vi "Gas Controller.vi"() -> ()   [LabVIEW 2013]
uses:
  Program Files/National Instruments/LabVIEW 2018/instr.lib/MultiGasController/647 Multi Gas Controller.llb/647 Open/Close Valve .vi
  <vilib>/MakerHub/LINX/LMH-LINX.lvlib
  <vilib>/MakerHub/LINX/Public/Sensors/Motion/Servo/Servo.lvlib
  <vilib>/Instr/_visa.llb/VISA Configure Serial Port (Instr).vi
  <vilib>/MakerHub/LINX/Public/Sensors/Motion/Servo/Servo Set Pulse Width One Channel.vi
  <vilib>/MakerHub/LINX/Public/Utilities/Open Serial.vi
  <vilib>/MakerHub/LINX/Public/Sensors/Motion/Servo/Servo Open One Channel.vi
  <vilib>/MakerHub/LINX/Public/Sensors/Motion/Servo/Servo Close One Channel.vi
  <vilib>/ErrorRing/Error Ring.xnode
  <vilib>/Utility/error.llb/Error Cluster From Error Code.vi
panel:
  out "MFC 8 Flow":dbl=-0.0
  out "MFC 7 Flow":dbl=-0.0
  out "MFC 6 Flow":dbl
  out "MFC 5 Flow":dbl=-0.094
  out "MFC 4 Flow":dbl=-0.303
  out "MFC 3 Flow":dbl=0.061
  out "MFC 2 Flow":dbl=-0.18
  out "MFC 1 Flow":dbl=10.022499999999999
  in  "Servo Channel":u8=11
  in  "On Position":dbl=860.0
  in  "Off Position":dbl=1900.0
  in  "Arduino Port":refnum<visa-resource-name>="COM7"
  in  "GCF 8":dbl=1.0
  in  "GCF 7":dbl=1.0
  in  "GCF 6":dbl=0.7
  in  "MFC 8 Size":dbl=1.0
  in  "MFC 7 Size":dbl=1.0
  in  "MFC 6 Size":dbl=50.0
  out "MFC 8 Status":bool
  out "MFC 7 Status":bool
  out "MFC 6 Status":bool
  in  "MFC 7":bool
  in  "MFC 8":bool
  in  "MFC 6: CO2":bool
  in  "MFC 8 set point":dbl
  in  "MFC 7 set point":dbl
  in  "MFC 6 set point":dbl
  in  "GCF 5":dbl=0.94
  in  "GCF 4":dbl=1.01
  in  "GCF 3":dbl=1.22
  in  "GCF 2":dbl=0.9
  in  "GCF 1":dbl=0.95
  in  "MFC 5 Size":dbl=100.0
  in  "MFC 4 Size":dbl=50.0
  in  "MFC 3 Size":dbl=50.0
  in  "MFC 2 Size":dbl=100.0
  in  "MFC 1 Size":dbl=50.0
  in  "stop":bool
  out "MFC 5 Status":bool
  out "MFC 4 Status":bool
  out "MFC 1 Status":bool=TRUE
  out "MFC 2 Status":bool
  out "MFC 3 Status":bool
  in  "MFC 2: N2":bool
  in  "MFC 2 set point":dbl=50.0
  in  "MFC 4: H2":bool
  in  "MFC 5: N2 (Wet)":bool
  in  "MFC 3: O2":bool
  in  "MFC 1: N2 to Microbalance":bool=TRUE
  in  "MFC 5 set point":dbl=48.5
  in  "MFC 4 set point":dbl=50.0
  in  "MFC 3 set point":dbl=50.0
  in  "MFC 1  set point":dbl=10.0
  in  "MKS Controller Port":refnum<visa-resource-name>="COM5"
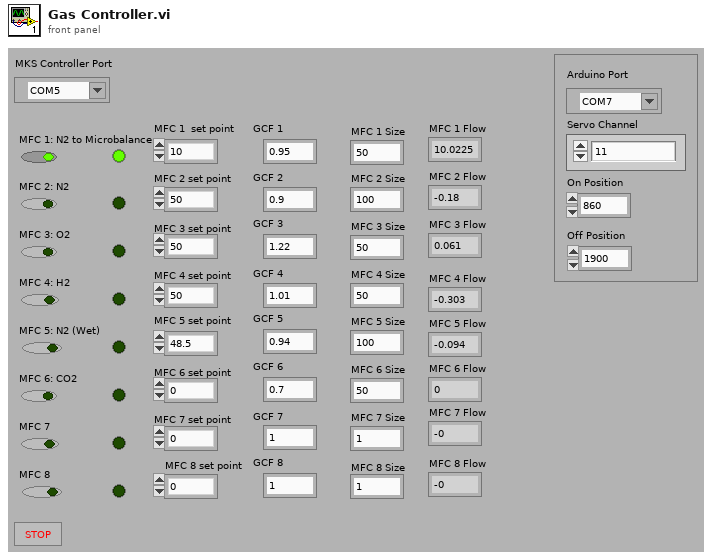
[diagram p1: front panel]
types:
  T1 = typedef "LMH-LINX.lvlib/LINX Ref.ctl" = cluster{"IO":T2, "Interface":T3, "LINX Device Config":T4}
  T2 = typedef "LMH-LINX.lvlib/Platform.ctl" = enum16{"Remote", "Local"}
  T3 = typedef "LMH-LINX.lvlib/Interface.ctl" = enum16{"Serial", "TCP"}
  T4 = typedef "LMH-LINX.lvlib/Device.lvlib/LINX Device Config.ctl" = cluster{"Interface":T3, "COM Port":refnum<visa-resource-name>, "TCP Configuration":T5, "Device Family":u8, "Device ID":u8, "Device Name":string, "TCP Ref":refnum<k5>, "Channels":T6}
  T5 = typedef "LMH-LINX.lvlib/Device.lvlib/TCP Config.ctl" = cluster{"IP Address":string, "Port":u16}
  T6 = typedef "LMH-LINX.lvlib/Channels.ctl" = cluster{"DI":u8[], "DO":u8[], "AI":u8[], "AO":u8[], "PWM":u8[], "QE":u8[], "UART":u8[], "I2C 2":u8[], "SPI":u8[], "CAN":u8[], "Servo":u8[], "AI Ref (V)":dbl, "AI Resolution (Bits)":u8, "AO Ref (V)":dbl, "AO Resolution (Bits)":u8}
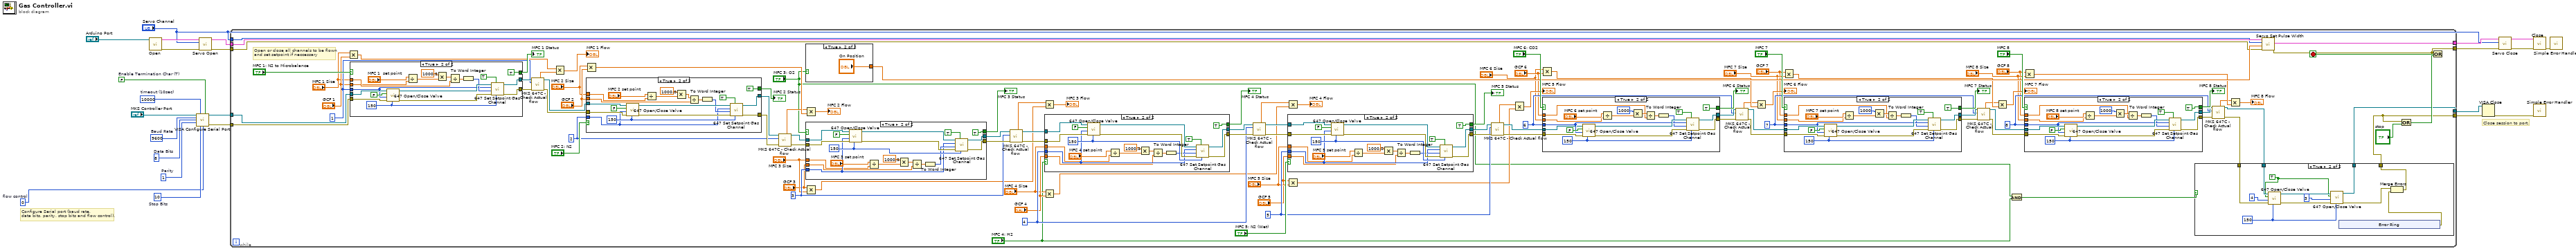
[diagram p0: block diagram]
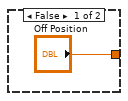
[diagram p3: hidden frame]
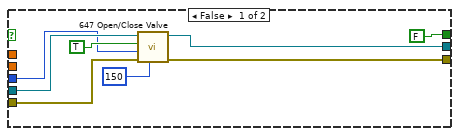
[diagram p4: hidden frame]
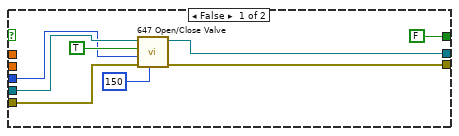
[diagram p5: hidden frame]
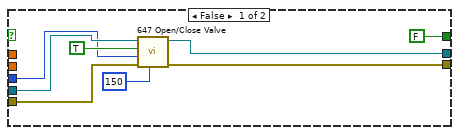
[diagram p6: hidden frame]
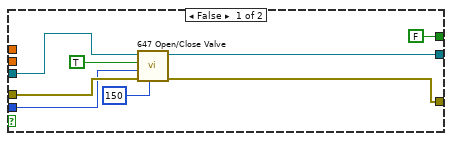
[diagram p7: hidden frame]
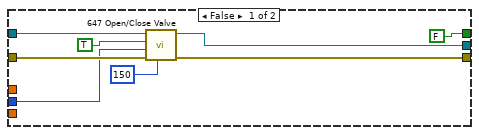
[diagram p8: hidden frame]
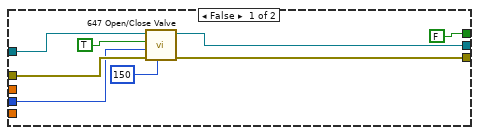
[diagram p9: hidden frame]
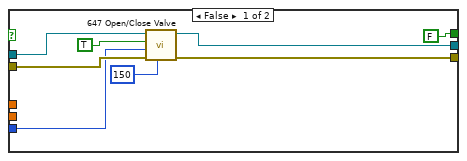
[diagram p10: hidden frame]
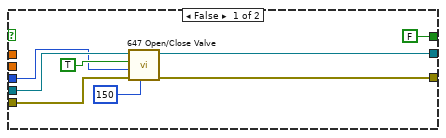
[diagram p11: hidden frame]
diagram:
  w17 = 0  # flow control
  w18 = 10  # Stop Bits
  w19 = 1  # Parity
  w20 = 8  # Data Bits
  w21 = 9600  # Baud Rate
  w22 = FALSE  # Enable Termination Char (T)
  w23 = u32 10000  # timeout (10sec)
  # "Close session to port."
  # "Configure Serial port (baud rate,\ndata bits, parity, stop bits and flow control)."
  n1 = call-poly <vilib>:"Open.vi"("Serial Port"="Arduino Port") -> ("Error Out"=w7:errorcluster, "LINX Resource"=w8:T1)  [unwired: 8 in, 1 out]
  n2 = call-poly "VISA Configure Serial Port"("VISA resource name"="MKS Controller Port", "timeout (10sec)"=w23, "Enable Termination\nChar (T)"=w22, "baud rate (9600)"=w21, "data bits (8)"=w20, "parity (0:none)"=w19, "stop bits (10: 1 bit)"=w18, "flow control (0:none)"=w17) -> ("VISA resource name out"=w16:refnum<visa-resource-name>, "error out"=w15:errorcluster)  [unwired: 6 in]
  n3 = call-poly <vilib>:"Servo Open.vi"("Error In"=w7, "Servo Channel"="Servo Channel", "LINX Resource"=w8) -> ("Error Out"=w4:errorcluster, "LINX Resource"=w5:T1)  [unwired: 7 in]
  n4 = while {
    tunnel: w16 -> [w126]
    tunnel: w15 -> [w125]
    tunnel: [w25] -> w13
    tunnel: [w26] -> w12
    tunnel: w5 -> [w117]
    tunnel: w4 -> [w116]
    tunnel: [w33] -> w3
    tunnel: [w115] -> w2
    tunnel: "Servo Channel" -> [w114]
    stop <- w35 stop-if-true
    w42 = 8
    w50 = 7
    w59 = 6
    w89 = 3
    w79 = 4
    w69 = 5
    w99 = 2
    w109 = 1
    # "Open or close all channels to be flown\nand set setpoint if neccessary"
    n5 = Multiply(x="MFC 1 Size", y="GCF 1") -> (x*y=w108:dbl)
    n6 = case shown="True" "MFC 1: N2 to Microbalance" {
      tunnel: w125 -> [w348 w371]
      tunnel: [w349 w366] -> w111
      tunnel: w126 -> [w351 w370]
      tunnel: [w350 w367] -> w113
      tunnel: w109 -> [w347 w357]
      tunnel: [FALSE TRUE] -> w129
      tunnel: "GCF 1" -> [_ w354]
      tunnel: "MFC 1 Size" -> [_ w353]
      frame False {
        n7 = call "647 Open/Close Valve .vi"("ms Wartezeit"=u32 150, "error in (no error)"=w348, "Channel number"=w347, "OPEN / CLOSE"=TRUE, "VISA session"=w351) -> ("error out"=w349:errorcluster, "dup VISA session"=w350:refnum<visa-resource-name>)  [unwired: 4 in, 1 out]
      }
      frame True {
        w364 = 150
        n8 = call "647 Open/Close Valve .vi"("ms Wartezeit"=w364, "error in (no error)"=w371, "Channel number"=w357, "OPEN / CLOSE"=FALSE, "VISA session"=w370) -> ("error out"=w365:errorcluster, "dup VISA session"=w368:refnum<visa-resource-name>)  [unwired: 4 in, 1 out]
        n9 = Divide(x="MFC 1  set point", y=w353) -> (x/y=w359:dbl)
        n10 = Multiply(x=1000.0, y=w359) -> (x*y=w358:dbl)
        n11 = Divide(x=w358, y=w354) -> (x/y=w355:dbl)
        n12 = To Word Integer(number=w355) -> (16bit integer=w362:i16)
        n13 = call "647 Set Setpoint Gas Channel.vi"("ms Wartezeit"=w364, "Read / Write"=TRUE, "error in (no error)"=w365, "Setpoint 0..1100\n0.1% F.S. MFC"=w362, "Channel number"=w357, "VISA session"=w368) -> ("error out"=w366:errorcluster, "dup VISA session"=w367:refnum<visa-resource-name>)  [unwired: 3 in, 1 out]
      }
    }
    "MFC 1 Status" <- w129
    n14 = call "MKS 647C - Check Actual flow.vi"("error in (no error)"=w111, "Channel"=w109, "VISA resource name (IN)"=w113) -> ("error out"=w110:errorcluster, "VISA resource name (OUT)"=w112:refnum<visa-resource-name>, "Flow value"=w106:dbl)  [unwired: 6 in]
    n15 = Multiply(x=w108, y=w106) -> (x*y=→"MFC 1 Flow":dbl)
    n16 = Multiply(x="MFC 2 Size", y="GCF 2") -> (x*y=w97:dbl)
    n17 = case shown="True" "MFC 2: N2" {
      tunnel: w112 -> [w242 w263]
      tunnel: w110 -> [w241 w262]
      tunnel: [w240 w259] -> w100
      tunnel: [w239 w258] -> w103
      tunnel: w99 -> [w238 w252]
      tunnel: [FALSE TRUE] -> w130
      tunnel: "MFC 2 Size" -> [_ w246]
      tunnel: "GCF 2" -> [_ w245]
      frame False {
        n18 = call "647 Open/Close Valve .vi"("ms Wartezeit"=u32 150, "error in (no error)"=w241, "Channel number"=w238, "OPEN / CLOSE"=TRUE, "VISA session"=w242) -> ("error out"=w240:errorcluster, "dup VISA session"=w239:refnum<visa-resource-name>)  [unwired: 4 in, 1 out]
      }
      frame True {
        w256 = 150
        n19 = call "647 Open/Close Valve .vi"("ms Wartezeit"=w256, "error in (no error)"=w262, "Channel number"=w252, "OPEN / CLOSE"=FALSE, "VISA session"=w263) -> ("error out"=w260:errorcluster, "dup VISA session"=w257:refnum<visa-resource-name>)  [unwired: 4 in, 1 out]
        n20 = Divide(x="MFC 2 set point", y=w246) -> (x/y=w251:dbl)
        n21 = Multiply(x=1000.0, y=w251) -> (x*y=w247:dbl)
        n22 = Divide(x=w247, y=w245) -> (x/y=w248:dbl)
        n23 = To Word Integer(number=w248) -> (16bit integer=w254:i16)
        n24 = call "647 Set Setpoint Gas Channel.vi"("ms Wartezeit"=w256, "Read / Write"=TRUE, "error in (no error)"=w260, "Setpoint 0..1100\n0.1% F.S. MFC"=w254, "Channel number"=w252, "VISA session"=w257) -> ("error out"=w259:errorcluster, "dup VISA session"=w258:refnum<visa-resource-name>)  [unwired: 3 in, 1 out]
      }
    }
    "MFC 2 Status" <- w130
    n25 = call "MKS 647C - Check Actual flow.vi"("error in (no error)"=w100, "Channel"=w99, "VISA resource name (IN)"=w103) -> ("error out"=w101:errorcluster, "VISA resource name (OUT)"=w102:refnum<visa-resource-name>, "Flow value"=w96:dbl)  [unwired: 6 in]
    n26 = Multiply(x=w96, y=w97) -> (x*y=→"MFC 2 Flow":dbl)
    n27 = Multiply(x="GCF 3", y="MFC 3 Size") -> (x*y=w87:dbl)
    n28 = case shown="True" "MFC 3: O2" {
      tunnel: ["Off Position" "On Position"] -> w118
      frame False {
      }
      frame True {
      }
    }
    n29 = case shown="True" "MFC 3: O2" {
      tunnel: w101 -> [w323 w344]
      tunnel: [w324 w338] -> w92
      tunnel: w102 -> [w322 w343]
      tunnel: [w325 w341] -> w91
      tunnel: w89 -> [w320 w332]
      tunnel: [FALSE TRUE] -> w131
      tunnel: "MFC 3 Size" -> [_ w327]
      tunnel: "GCF 3" -> [_ w326]
      frame False {
        n30 = call "647 Open/Close Valve .vi"("ms Wartezeit"=u32 150, "error in (no error)"=w323, "Channel number"=w320, "OPEN / CLOSE"=TRUE, "VISA session"=w322) -> ("error out"=w324:errorcluster, "dup VISA session"=w325:refnum<visa-resource-name>)  [unwired: 4 in, 1 out]
      }
      frame True {
        w337 = 150
        n31 = call "647 Open/Close Valve .vi"("ms Wartezeit"=w337, "error in (no error)"=w344, "Channel number"=w332, "OPEN / CLOSE"=FALSE, "VISA session"=w343) -> ("error out"=w339:errorcluster, "dup VISA session"=w340:refnum<visa-resource-name>)  [unwired: 4 in, 1 out]
        n32 = Divide(x="MFC 3 set point", y=w327) -> (x/y=w335:dbl)
        n33 = Multiply(x=1000.0, y=w335) -> (x*y=w328:dbl)
        n34 = Divide(x=w328, y=w326) -> (x/y=w329:dbl)
        n35 = To Word Integer(number=w329) -> (16bit integer=w334:i16)
        n36 = call "647 Set Setpoint Gas Channel.vi"("ms Wartezeit"=w337, "Read / Write"=TRUE, "error in (no error)"=w339, "Setpoint 0..1100\n0.1% F.S. MFC"=w334, "Channel number"=w332, "VISA session"=w340) -> ("error out"=w338:errorcluster, "dup VISA session"=w341:refnum<visa-resource-name>)  [unwired: 3 in, 1 out]
      }
    }
    "MFC 3 Status" <- w131
    n37 = call "MKS 647C - Check Actual flow.vi"("error in (no error)"=w92, "Channel"=w89, "VISA resource name (IN)"=w91) -> ("error out"=w93:errorcluster, "VISA resource name (OUT)"=w90:refnum<visa-resource-name>, "Flow value"=w84:dbl)  [unwired: 6 in]
    n38 = Multiply(x=w84, y=w87) -> (x*y=→"MFC 3 Flow":dbl)
    n39 = Multiply(x="MFC 4 Size", y="GCF 4") -> (x*y=w77:dbl)
    n40 = case shown="True" "MFC 4: H2" {
      tunnel: w93 -> [w298 w316]
      tunnel: [w297 w312] -> w81
      tunnel: w90 -> [w296 w317]
      tunnel: [w295 w313] -> w80
      tunnel: [FALSE TRUE] -> w128
      tunnel: w79 -> [w291 w303]
      tunnel: "MFC 4 Size" -> [_ w300]
      tunnel: "GCF 4" -> [_ w299]
      frame False {
        n41 = call "647 Open/Close Valve .vi"("ms Wartezeit"=u32 150, "error in (no error)"=w298, "Channel number"=w291, "OPEN / CLOSE"=TRUE, "VISA session"=w296) -> ("error out"=w297:errorcluster, "dup VISA session"=w295:refnum<visa-resource-name>)  [unwired: 4 in, 1 out]
      }
      frame True {
        w310 = u32 150
        n42 = call "647 Open/Close Valve .vi"("ms Wartezeit"=w310, "error in (no error)"=w316, "Channel number"=w303, "OPEN / CLOSE"=FALSE, "VISA session"=w317) -> ("error out"=w311:errorcluster, "dup VISA session"=w314:refnum<visa-resource-name>)  [unwired: 4 in, 1 out]
        n43 = Divide(x="MFC 4 set point", y=w300) -> (x/y=w308:dbl)
        n44 = Multiply(x=1000.0, y=w308) -> (x*y=w301:dbl)
        n45 = Divide(x=w301, y=w299) -> (x/y=w302:dbl)
        n46 = To Word Integer(number=w302) -> (16bit integer=w307:i16)
        n47 = call "647 Set Setpoint Gas Channel.vi"("ms Wartezeit"=w310, "Read / Write"=TRUE, "error in (no error)"=w311, "Setpoint 0..1100\n0.1% F.S. MFC"=w307, "Channel number"=w303, "VISA session"=w314) -> ("error out"=w312:errorcluster, "dup VISA session"=w313:refnum<visa-resource-name>)  [unwired: 3 in, 1 out]
      }
    }
    "MFC 4 Status" <- w128
    n48 = call "MKS 647C - Check Actual flow.vi"("error in (no error)"=w81, "Channel"=w79, "VISA resource name (IN)"=w80) -> ("error out"=w82:errorcluster, "VISA resource name (OUT)"=w83:refnum<visa-resource-name>, "Flow value"=w74:dbl)  [unwired: 6 in]
    n49 = Multiply(x=w74, y=w77) -> (x*y=→"MFC 4 Flow":dbl)
    n50 = Multiply(x="GCF 5", y="MFC 5 Size") -> (x*y=w67:dbl)
    n51 = case shown="True" "MFC 5: N2 (Wet)" {
      tunnel: w82 -> [w271 w289]
      tunnel: w83 -> [w270 w290]
      tunnel: [FALSE TRUE] -> w127
      tunnel: w69 -> [w266 w278]
      tunnel: [w264 w275] -> w73
      tunnel: [w265 w274] -> w70
      tunnel: "GCF 5" -> [_ w273]
      tunnel: "MFC 5 Size" -> [_ w272]
      frame False {
        n52 = call "647 Open/Close Valve .vi"("ms Wartezeit"=u32 150, "error in (no error)"=w271, "Channel number"=w266, "OPEN / CLOSE"=TRUE, "VISA session"=w270) -> ("error out"=w265:errorcluster, "dup VISA session"=w264:refnum<visa-resource-name>)  [unwired: 4 in, 1 out]
      }
      frame True {
        w285 = u32 150
        n53 = call "647 Open/Close Valve .vi"("ms Wartezeit"=w285, "error in (no error)"=w289, "Channel number"=w278, "OPEN / CLOSE"=FALSE, "VISA session"=w290) -> ("error out"=w286:errorcluster, "dup VISA session"=w287:refnum<visa-resource-name>)  [unwired: 4 in, 1 out]
        n54 = Divide(x="MFC 5 set point", y=w272) -> (x/y=w283:dbl)
        n55 = Multiply(x=1000.0, y=w283) -> (x*y=w277:dbl)
        n56 = Divide(x=w277, y=w273) -> (x/y=w276:dbl)
        n57 = To Word Integer(number=w276) -> (16bit integer=w282:i16)
        n58 = call "647 Set Setpoint Gas Channel.vi"("ms Wartezeit"=w285, "Read / Write"=TRUE, "error in (no error)"=w286, "Setpoint 0..1100\n0.1% F.S. MFC"=w282, "Channel number"=w278, "VISA session"=w287) -> ("error out"=w274:errorcluster, "dup VISA session"=w275:refnum<visa-resource-name>)  [unwired: 3 in, 1 out]
      }
    }
    "MFC 5 Status" <- w127
    n59 = call "MKS 647C - Check Actual flow.vi"("error in (no error)"=w70, "Channel"=w69, "VISA resource name (IN)"=w73) -> ("error out"=w71:errorcluster, "VISA resource name (OUT)"=w72:refnum<visa-resource-name>, "Flow value"=w66:dbl)  [unwired: 6 in]
    n60 = Multiply(x=w66, y=w67) -> (x*y=→"MFC 5 Flow":dbl)
    n61 = Multiply(x="MFC 6 Size", y="GCF 6") -> (x*y=w58:dbl)
    n62 = case shown="True" "MFC 6: CO2" {
      tunnel: [FALSE TRUE] -> w123
      tunnel: [w216 w231] -> w61
      tunnel: [w214 w230] -> w60
      tunnel: w59 -> [w212 w229]
      tunnel: w72 -> [w215 w227]
      tunnel: w71 -> [w217 w226]
      tunnel: "GCF 6" -> [_ w219]
      tunnel: "MFC 6 Size" -> [_ w218]
      frame False {
        n63 = call "647 Open/Close Valve .vi"("ms Wartezeit"=150, "error in (no error)"=w217, "Channel number"=w212, "OPEN / CLOSE"=TRUE, "VISA session"=w215) -> ("error out"=w216:errorcluster, "dup VISA session"=w214:refnum<visa-resource-name>)  [unwired: 4 in, 1 out]
      }
      frame True {
        w228 = 150
        n64 = call "647 Open/Close Valve .vi"("ms Wartezeit"=w228, "error in (no error)"=w226, "Channel number"=w229, "OPEN / CLOSE"=FALSE, "VISA session"=w227) -> ("error out"=w234:errorcluster, "dup VISA session"=w233:refnum<visa-resource-name>)  [unwired: 4 in, 1 out]
        n65 = Divide(x="MFC 6 set point", y=w218) -> (x/y=w224:dbl)
        n66 = Multiply(x=1000, y=w224) -> (x*y=w220:dbl)
        n67 = Divide(x=w220, y=w219) -> (x/y=w222:dbl)
        n68 = To Word Integer(number=w222) -> (16bit integer=w221:i16)
        n69 = call "647 Set Setpoint Gas Channel.vi"("ms Wartezeit"=w228, "Read / Write"=TRUE, "error in (no error)"=w234, "Setpoint 0..1100\n0.1% F.S. MFC"=w221, "Channel number"=w229, "VISA session"=w233) -> ("error out"=w231:errorcluster, "dup VISA session"=w230:refnum<visa-resource-name>)  [unwired: 3 in, 1 out]
      }
    }
    "MFC 6 Status" <- w123
    n70 = call "MKS 647C - Check Actual flow.vi"("error in (no error)"=w61, "Channel"=w59, "VISA resource name (IN)"=w60) -> ("error out"=w62:errorcluster, "VISA resource name (OUT)"=w63:refnum<visa-resource-name>, "Flow value"=w54:dbl)  [unwired: 6 in]
    n71 = Multiply(x=w54, y=w58) -> (x*y=→"MFC 6 Flow":dbl)
    n72 = Multiply(x="GCF 7", y="MFC 7 Size") -> (x*y=w49:dbl)
    n73 = case shown="True" "MFC 7" {
      tunnel: [FALSE TRUE] -> w122
      tunnel: w62 -> [w190 w204]
      tunnel: [w189 w203] -> w51
      tunnel: w63 -> [w188 w202]
      tunnel: [w187 w201] -> w53
      tunnel: w50 -> [w185 w200]
      tunnel: "MFC 7 Size" -> [_ w192]
      tunnel: "GCF 7" -> [_ w191]
      frame False {
        n74 = call "647 Open/Close Valve .vi"("ms Wartezeit"=150, "error in (no error)"=w190, "Channel number"=w185, "OPEN / CLOSE"=TRUE, "VISA session"=w188) -> ("error out"=w189:errorcluster, "dup VISA session"=w187:refnum<visa-resource-name>)  [unwired: 4 in, 1 out]
      }
      frame True {
        w199 = 150
        n75 = call "647 Open/Close Valve .vi"("ms Wartezeit"=w199, "error in (no error)"=w204, "Channel number"=w200, "OPEN / CLOSE"=FALSE, "VISA session"=w202) -> ("error out"=w207:errorcluster, "dup VISA session"=w208:refnum<visa-resource-name>)  [unwired: 4 in, 1 out]
        n76 = Divide(x="MFC 7 set point", y=w192) -> (x/y=w197:dbl)
        n77 = Multiply(x=1000, y=w197) -> (x*y=w193:dbl)
        n78 = Divide(x=w193, y=w191) -> (x/y=w195:dbl)
        n79 = To Word Integer(number=w195) -> (16bit integer=w194:i16)
        n80 = call "647 Set Setpoint Gas Channel.vi"("ms Wartezeit"=w199, "Read / Write"=TRUE, "error in (no error)"=w207, "Setpoint 0..1100\n0.1% F.S. MFC"=w194, "Channel number"=w200, "VISA session"=w208) -> ("error out"=w203:errorcluster, "dup VISA session"=w201:refnum<visa-resource-name>)  [unwired: 3 in, 1 out]
      }
    }
    "MFC 7 Status" <- w122
    n81 = call "MKS 647C - Check Actual flow.vi"("error in (no error)"=w51, "Channel"=w50, "VISA resource name (IN)"=w53) -> ("error out"=w52:errorcluster, "VISA resource name (OUT)"=w29:refnum<visa-resource-name>, "Flow value"=w46:dbl)  [unwired: 6 in]
    n82 = Multiply(x=w46, y=w49) -> (x*y=→"MFC 7 Flow":dbl)
    n83 = And(x="MFC 3: O2", y="MFC 4: H2") -> (x .and. y?=w32:bool)
    n84 = Multiply(x="GCF 8", y="MFC 8 Size") -> (x*y=w41:dbl)
    n85 = case shown="True" "MFC 8" {
      tunnel: [FALSE TRUE] -> w121
      tunnel: w52 -> [w163 w177]
      tunnel: w29 -> [w161 w176]
      tunnel: w42 -> [w158 w175]
      tunnel: [w162 w173] -> w44
      tunnel: [w160 w167] -> w43
      tunnel: "MFC 8 Size" -> [_ w165]
      tunnel: "GCF 8" -> [_ w164]
      frame False {
        n86 = call "647 Open/Close Valve .vi"("ms Wartezeit"=150, "error in (no error)"=w163, "Channel number"=w158, "OPEN / CLOSE"=TRUE, "VISA session"=w161) -> ("error out"=w162:errorcluster, "dup VISA session"=w160:refnum<visa-resource-name>)  [unwired: 4 in, 1 out]
      }
      frame True {
        w174 = 150
        n87 = call "647 Open/Close Valve .vi"("ms Wartezeit"=w174, "error in (no error)"=w177, "Channel number"=w175, "OPEN / CLOSE"=FALSE, "VISA session"=w176) -> ("error out"=w180:errorcluster, "dup VISA session"=w181:refnum<visa-resource-name>)  [unwired: 4 in, 1 out]
        n88 = Divide(x="MFC 8 set point", y=w165) -> (x/y=w171:dbl)
        n89 = Multiply(x=1000, y=w171) -> (x*y=w166:dbl)
        n90 = Divide(x=w166, y=w164) -> (x/y=w169:dbl)
        n91 = To Word Integer(number=w169) -> (16bit integer=w168:i16)
        n92 = call "647 Set Setpoint Gas Channel.vi"("ms Wartezeit"=w174, "Read / Write"=TRUE, "error in (no error)"=w180, "Setpoint 0..1100\n0.1% F.S. MFC"=w168, "Channel number"=w175, "VISA session"=w181) -> ("error out"=w173:errorcluster, "dup VISA session"=w167:refnum<visa-resource-name>)  [unwired: 3 in, 1 out]
      }
    }
    "MFC 8 Status" <- w121
    n93 = call "MKS 647C - Check Actual flow.vi"("error in (no error)"=w44, "Channel"=w42, "VISA resource name (IN)"=w43) -> ("error out"=w28:errorcluster, "VISA resource name (OUT)"=w27:refnum<visa-resource-name>, "Flow value"=w37:dbl)  [unwired: 6 in]
    n94 = case shown="True" w32 {
      tunnel: w27 -> [w136 w146]
      tunnel: [w136 w145] -> w26
      tunnel: [w135 w137] -> w25
      tunnel: w28 -> [w135 w144]
      frame False {
      }
      frame True {
        w142 = TRUE
        w143 = 150
        n95 = call "647 Open/Close Valve .vi"("ms Wartezeit"=w143, "error in (no error)"=w144, "Channel number"=4, "OPEN / CLOSE"=w142, "VISA session"=w146) -> ("error out"=w148:errorcluster, "dup VISA session"=w147:refnum<visa-resource-name>)  [unwired: 4 in, 1 out]
        n96 = call "647 Open/Close Valve .vi"("ms Wartezeit"=w143, "error in (no error)"=w148, "Channel number"=3, "OPEN / CLOSE"=w142, "VISA session"=w147) -> ("error out"=w138:errorcluster, "dup VISA session"=w145:refnum<visa-resource-name>)  [unwired: 4 in, 1 out]
        n97 = xnode "Error Ring"() -> ("error out"=w139:errorcluster)
        n98 = Merge Errors(w138, w139) -> (w137:errorcluster)
      }
    }
    n99 = Multiply(x=w37, y=w41) -> (x*y=→"MFC 8 Flow":dbl)
    n100 = call-poly <vilib>:"Servo Set Pulse Width.vi"("Error In"=w116, "Pulse Width (uS)"=w118, "Servo Channel"=w114, "LINX Resource"=w117) -> ("Error Out"=w33:errorcluster, "LINX Resource"=w115:T1)  [unwired: 6 in]
    n101 = Or(x=w25, y="stop") -> (x .or. y?=w34:bool)
    n102 = Or(x=w33, y=w34) -> (x .or. y?=w35:bool)
  }
  n103 = VISA Close(VISA resource name=w12, error in (no error)=w13) -> (error out=w14:errorcluster)
  n104 = call-poly <vilib>:"Servo Close.vi"("Error In"=w3, "Servo Channel"="Servo Channel", "LINX Resource"=w2) -> ("Error Out"=w11:errorcluster, "LINX Resource"=w10:T1)  [unwired: 7 in]
  n105 = call <vilib>:"Close.vi"("Error In"=w11, "LINX Resource"=w10) -> ("Error Out"=w9:errorcluster)  [unwired: 9 in]
  n106 = call <vilib>:"Simple Error Handler.vi"("error in (no error)"=w14) -> ()  [unwired: 4 in, 5 out]
  n107 = call <vilib>:"Simple Error Handler.vi"("error in (no error)"=w9) -> ()  [unwired: 4 in, 5 out]
